vi "day 5 task 1.vi"() -> ()   [LabVIEW 2019]
panel:
  out "String":string
  out "Array 3":string[][](array[string])
  out "output array":string[][](array[string])
  out "Array":string[][](array[string])
  out "Array 2":string[][](array[string])
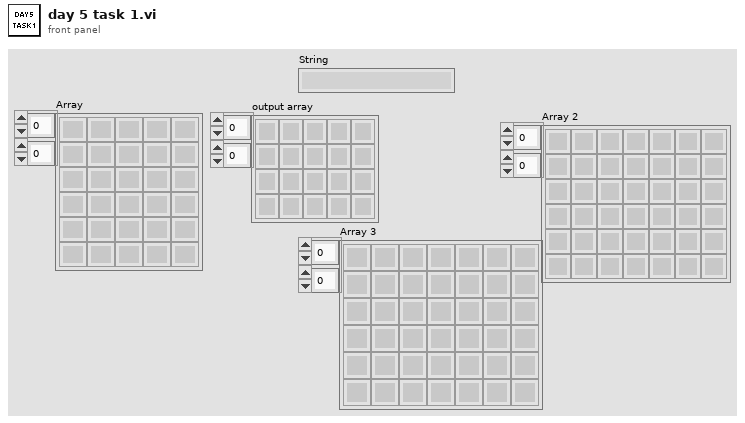
[diagram p1: front panel]
types:
  T1 = cluster{"no. crates to move":i32, "source col index":i32, "destination col index":i32}
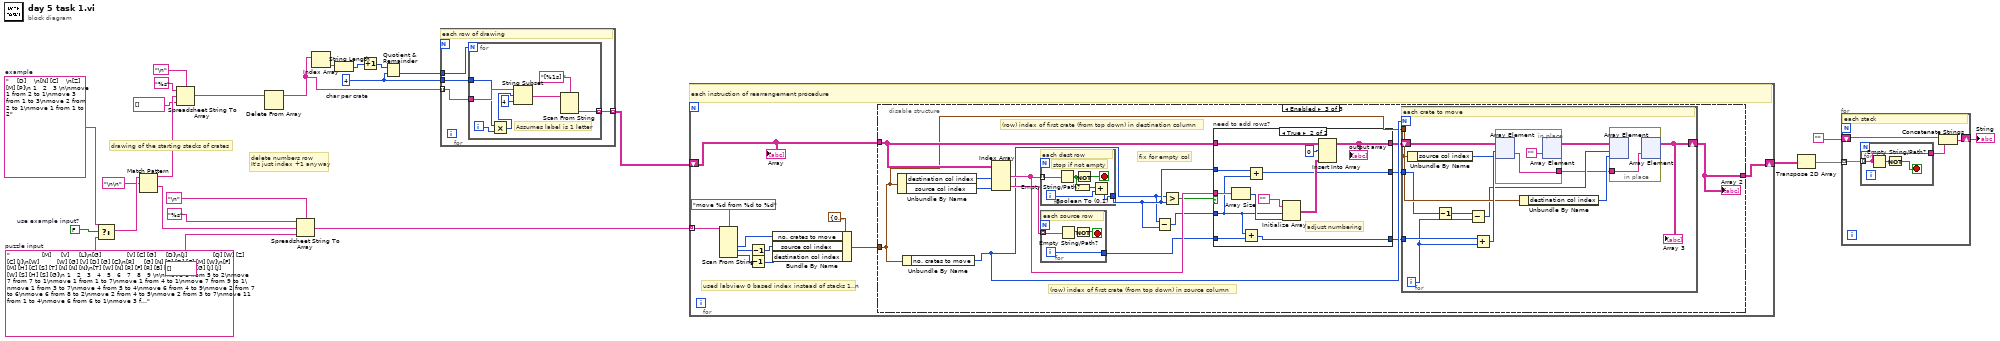
[diagram p0: block diagram]
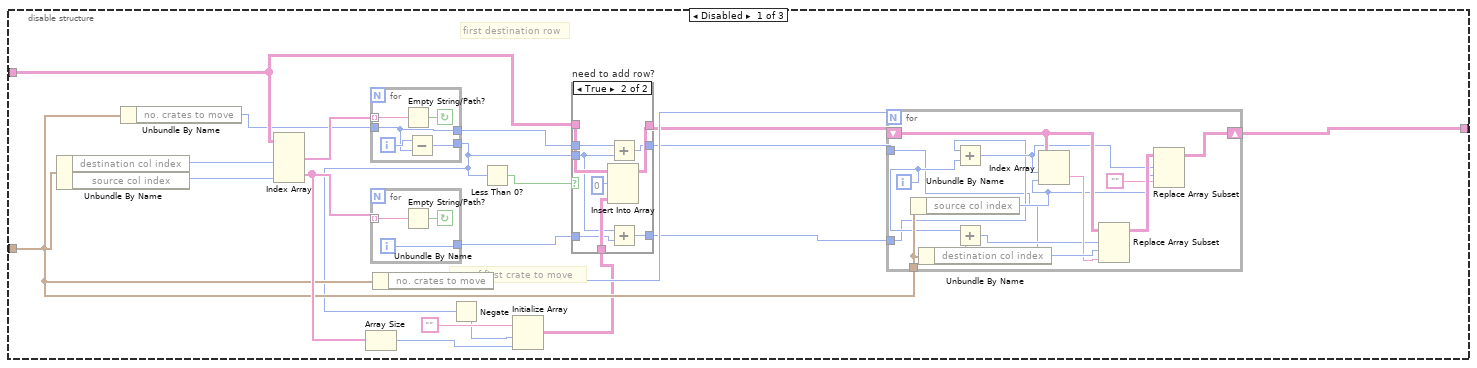
[diagram p2: hidden frame]
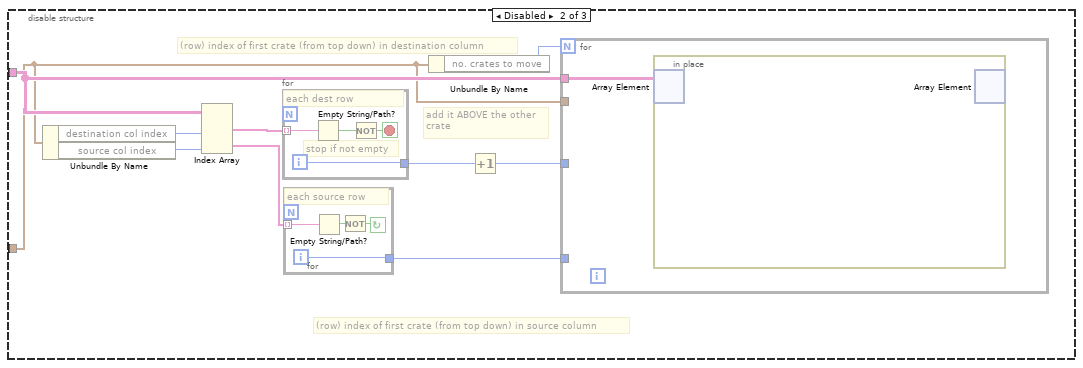
[diagram p4: hidden frame]
diagram:
  w11 = 4  # char per crate
  w21 = FALSE  # use example input?
  w22 = "                [M]     [V]     [L]\n[G]             [V] [C] [G]     [D]\n[J]             [Q] [W] [Z] [C] [J]\n[W]         [W] [G] [V] [D] [G] [C]\n[R]     [G] [N] [B] [D] [C] [M] [W]\n[F] [M] [H] [C] [S] [T] [N] [N] [N]\n[T] [W] [N] [R] [F] [R] [B] [J] [P]\n[Z] [G] [J] [J] [W] [S] [H] [S] [G]\n 1   2   3   4   5   6   7   8   9 \n\nmove 1 from 5 to 2\nmove 7 from 7 to 1\nmove 1 from 1 to 7\nmove 1 from 4 to 1\nmove 7 from 9 to 1\nmove 1 from 3 to 7\nmove 4 from 5 to 4\nmove 6 from 4 to 9\nmove 2 from 7 to 6\nmove 6 from 8 to 2\nmove 2 from 4 to 5\nmove 2 from 3 to 7\nmove 11 from 1 to 4\nmove 6 from 6 to 1\nmove 3 from 5 to 3\nmove 5 from 9 to 8\nmove 1 from 2 to 3\nmove 2 from 7 to 9\nmove 7 from 1 to 2\nmove 1 from 5 to 3\nmove 1 from 5 to 3\nmove 5 from 8 to 5\nmove 3 from 5 to 4\nmove 1 from 1 to 7\nmove 1 from 3 to 8\nmove 2 from 6 to 3\nmove 3 from 3 to 4\nmove 1 from 6 to 2\nmove 5 from 4 to 2\nmove 2 from 5 to 3\nmove 2 from 7 to 1\nmove 1 from 8 to 1\nmove 7 from 1 to 7\nmove 4 from 4 to 2\nmove 7 from 4 to 1\nmove 10 from 1 to 5\nmove 10 from 5 to 2\nmove 11 from 2 to 3\nmove 1 from 1 to 6\nmove 1 from 4 to 7\nmove 4 from 7 to 1\nmove 6 from 2 to 5\nmove 2 from 1 to 3\nmove 1 from 9 to 5\nmove 2 from 9 to 6\nmove 1 from 6 to 1\nmove 3 from 5 to 4\nmove 20 from 3 to 9\nmove 3 from 7 to 1\nmove 3 from 5 to 2\nmove 3 from 4 to 8\nmove 3 from 1 to 3\nmove 3 from 1 to 2\nmove 2 from 6 to 1\nmove 10 from 9 to 6\nmove 6 from 6 to 7\nmove 4 from 6 to 3\nmove 11 from 2 to 6\nmove 1 from 8 to 9\nmove 13 from 2 to 3\nmove 1 from 1 to 9\nmove 1 from 9 to 4\nmove 1 from 8 to 2\nmove 1 from 8 to 2\nmove 4 from 7 to 8\nmove 8 from 6 to 9\nmove 3 from 2 to 3\nmove 3 from 8 to 4\nmove 11 from 9 to 2\nmove 7 from 9 to 6\nmove 1 from 1 to 5\nmove 4 from 4 to 9\nmove 21 from 3 to 1\nmove 1 from 3 to 9\nmove 7 from 6 to 3\nmove 6 from 1 to 2\nmove 13 from 1 to 5\nmove 2 from 1 to 2\nmove 3 from 9 to 3\nmove 2 from 2 to 3\nmove 2 from 6 to 4\nmove 3 from 3 to 5\nmove 13 from 5 to 2\nmove 5 from 3 to 4\nmove 2 from 7 to 9\nmove 2 from 4 to 2\nmove 1 from 3 to 8\nmove 1 from 6 to 1\nmove 4 from 3 to 7\nmove 2 from 5 to 7\nmove 1 from 7 to 2\nmove 1 from 5 to 9\nmove 4 from 7 to 8\nmove 1 from 1 to 9\nmove 6 from 8 to 1\nmove 4 from 4 to 8\nmove 25 from 2 to 9\nmove 1 from 4 to 3\nmove 1 from 3 to 7\nmove 4 from 8 to 1\nmove 1 from 7 to 4\nmove 3 from 1 to 6\nmove 5 from 2 to 1\nmove 1 from 5 to 1\nmove 1 from 4 to 1\nmove 24 from 9 to 6\nmove 9 from 1 to 6\nmove 1 from 5 to 6\nmove 1 from 1 to 9\nmove 1 from 2 to 8\nmove 1 from 8 to 1\nmove 3 from 1 to 8\nmove 36 from 6 to 3\nmove 2 from 7 to 3\nmove 1 from 2 to 5\nmove 1 from 5 to 2\nmove 1 from 6 to 2\nmove 10 from 3 to 2\nmove 3 from 8 to 2\nmove 1 from 1 to 7\nmove 2 from 2 to 6\nmove 10 from 9 to 1\nmove 2 from 6 to 4\nmove 13 from 3 to 4\nmove 8 from 3 to 7\nmove 8 from 1 to 2\nmove 5 from 3 to 8\nmove 3 from 1 to 9\nmove 1 from 7 to 1\nmove 7 from 4 to 5\nmove 1 from 1 to 2\nmove 14 from 2 to 6\nmove 2 from 7 to 2\nmove 8 from 4 to 8\nmove 3 from 7 to 9\nmove 2 from 9 to 8\nmove 2 from 7 to 1\nmove 1 from 7 to 8\nmove 1 from 6 to 8\nmove 1 from 9 to 3\nmove 4 from 2 to 7\nmove 6 from 6 to 1\nmove 3 from 1 to 9\nmove 1 from 1 to 7\nmove 6 from 5 to 6\nmove 1 from 5 to 2\nmove 1 from 6 to 8\nmove 5 from 7 to 5\nmove 1 from 2 to 9\nmove 2 from 3 to 4\nmove 9 from 8 to 4\nmove 8 from 4 to 8\nmove 6 from 6 to 7\nmove 5 from 6 to 4\nmove 7 from 9 to 7\nmove 7 from 8 to 7\nmove 5 from 8 to 4\nmove 3 from 1 to 6\nmove 1 from 2 to 7\nmove 1 from 1 to 4\nmove 4 from 5 to 2\nmove 2 from 6 to 9\nmove 1 from 3 to 7\nmove 1 from 5 to 1\nmove 1 from 8 to 9\nmove 1 from 6 to 1\nmove 1 from 2 to 7\nmove 2 from 8 to 1\nmove 2 from 1 to 8\nmove 3 from 2 to 4\nmove 1 from 6 to 1\nmove 17 from 4 to 1\nmove 3 from 2 to 7\nmove 13 from 7 to 8\nmove 1 from 2 to 6\nmove 14 from 1 to 4\nmove 2 from 8 to 5\nmove 1 from 9 to 7\nmove 2 from 5 to 4\nmove 1 from 9 to 3\nmove 5 from 1 to 5\nmove 3 from 4 to 1\nmove 1 from 3 to 2\nmove 7 from 4 to 5\nmove 9 from 7 to 8\nmove 5 from 4 to 2\nmove 1 from 1 to 3\nmove 1 from 9 to 2\nmove 15 from 8 to 6\nmove 1 from 3 to 7\nmove 11 from 6 to 5\nmove 1 from 4 to 8\nmove 3 from 1 to 7\nmove 5 from 7 to 5\nmove 27 from 5 to 1\nmove 8 from 8 to 4\nmove 1 from 2 to 6\nmove 3 from 6 to 1\nmove 9 from 1 to 5\nmove 5 from 5 to 7\nmove 2 from 2 to 1\nmove 2 from 5 to 4\nmove 6 from 7 to 6\nmove 1 from 5 to 2\nmove 1 from 7 to 8\nmove 4 from 6 to 8\nmove 5 from 6 to 3\nmove 1 from 7 to 1\nmove 5 from 4 to 3\nmove 6 from 8 to 2\nmove 1 from 7 to 8\nmove 2 from 8 to 9\nmove 10 from 3 to 5\nmove 9 from 5 to 2\nmove 3 from 4 to 8\nmove 1 from 5 to 7\nmove 2 from 9 to 7\nmove 2 from 8 to 3\nmove 1 from 3 to 8\nmove 19 from 1 to 7\nmove 4 from 2 to 7\nmove 2 from 4 to 3\nmove 3 from 3 to 2\nmove 2 from 8 to 3\nmove 2 from 5 to 8\nmove 1 from 2 to 3\nmove 2 from 8 to 3\nmove 5 from 2 to 5\nmove 9 from 7 to 5\nmove 13 from 5 to 9\nmove 7 from 2 to 6\nmove 2 from 6 to 9\nmove 1 from 2 to 1\nmove 5 from 6 to 7\nmove 1 from 5 to 7\nmove 6 from 1 to 2\nmove 5 from 3 to 6\nmove 6 from 7 to 2\nmove 3 from 6 to 4\nmove 3 from 7 to 4\nmove 12 from 7 to 6\nmove 5 from 4 to 1\nmove 2 from 7 to 4\nmove 3 from 4 to 6\nmove 16 from 6 to 3\nmove 4 from 1 to 4\nmove 1 from 1 to 9\nmove 3 from 9 to 2\nmove 1 from 4 to 6\nmove 9 from 3 to 7\nmove 2 from 6 to 3\nmove 3 from 3 to 9\nmove 15 from 2 to 7\nmove 19 from 7 to 4\nmove 15 from 9 to 2\nmove 16 from 2 to 8\nmove 6 from 3 to 5\nmove 4 from 7 to 5\nmove 15 from 8 to 7\nmove 19 from 4 to 2\nmove 1 from 8 to 3\nmove 16 from 2 to 1\nmove 9 from 7 to 6\nmove 7 from 2 to 8\nmove 2 from 2 to 7\nmove 1 from 9 to 5\nmove 1 from 3 to 4\nmove 6 from 1 to 2\nmove 8 from 5 to 1\nmove 1 from 5 to 1\nmove 18 from 1 to 8\nmove 7 from 7 to 5\nmove 7 from 5 to 3\nmove 4 from 3 to 6\nmove 13 from 8 to 5\nmove 12 from 8 to 1\nmove 5 from 1 to 6\nmove 15 from 5 to 4\nmove 1 from 1 to 6\nmove 12 from 6 to 3\nmove 8 from 3 to 4\nmove 2 from 7 to 3\nmove 9 from 3 to 1\nmove 5 from 2 to 9\nmove 16 from 4 to 3\nmove 10 from 1 to 3\nmove 2 from 1 to 5\nmove 1 from 3 to 1\nmove 5 from 6 to 1\nmove 4 from 9 to 3\nmove 1 from 2 to 8\nmove 1 from 8 to 1\nmove 1 from 9 to 8\nmove 2 from 5 to 9\nmove 9 from 4 to 1\nmove 3 from 1 to 3\nmove 2 from 6 to 8\nmove 3 from 8 to 5\nmove 2 from 1 to 5\nmove 2 from 9 to 8\nmove 1 from 8 to 6\nmove 2 from 5 to 3\nmove 19 from 3 to 1\nmove 2 from 4 to 2\nmove 1 from 5 to 6\nmove 2 from 2 to 3\nmove 1 from 8 to 6\nmove 8 from 3 to 9\nmove 6 from 3 to 7\nmove 2 from 6 to 2\nmove 1 from 6 to 1\nmove 1 from 1 to 8\nmove 1 from 8 to 9\nmove 1 from 7 to 3\nmove 19 from 1 to 5\nmove 21 from 5 to 2\nmove 13 from 2 to 6\nmove 13 from 1 to 8\nmove 7 from 9 to 7\nmove 2 from 9 to 2\nmove 10 from 8 to 3\nmove 1 from 1 to 6\nmove 10 from 2 to 4\nmove 11 from 3 to 5\nmove 8 from 5 to 6\nmove 1 from 3 to 7\nmove 2 from 8 to 6\nmove 2 from 2 to 8\nmove 3 from 7 to 6\nmove 2 from 8 to 6\nmove 1 from 1 to 2\nmove 24 from 6 to 5\nmove 2 from 3 to 8\nmove 1 from 8 to 6\nmove 7 from 7 to 9\nmove 4 from 6 to 9\nmove 1 from 8 to 9\nmove 21 from 5 to 9\nmove 2 from 7 to 2\nmove 1 from 8 to 5\nmove 1 from 7 to 3\nmove 12 from 9 to 6\nmove 6 from 6 to 3\nmove 12 from 9 to 4\nmove 4 from 5 to 6\nmove 13 from 4 to 2\nmove 8 from 4 to 8\nmove 10 from 6 to 8\nmove 11 from 8 to 9\nmove 4 from 8 to 4\nmove 2 from 4 to 3\nmove 8 from 3 to 8\nmove 2 from 6 to 8\nmove 1 from 3 to 8\nmove 6 from 2 to 4\nmove 1 from 4 to 8\nmove 1 from 9 to 7\nmove 13 from 8 to 4\nmove 1 from 7 to 1\nmove 1 from 1 to 4\nmove 8 from 4 to 7\nmove 3 from 5 to 7\nmove 19 from 9 to 7\nmove 3 from 2 to 7\nmove 1 from 8 to 2\nmove 13 from 7 to 6\nmove 1 from 2 to 4\nmove 4 from 6 to 2\nmove 1 from 8 to 3\nmove 7 from 6 to 8\nmove 1 from 6 to 2\nmove 1 from 2 to 7\nmove 9 from 2 to 3\nmove 1 from 6 to 2\nmove 21 from 7 to 5\nmove 9 from 5 to 3\nmove 19 from 3 to 9\nmove 5 from 8 to 5\nmove 2 from 2 to 1\nmove 2 from 1 to 8\nmove 6 from 4 to 5\nmove 3 from 8 to 7\nmove 15 from 9 to 2\nmove 2 from 2 to 5\nmove 3 from 9 to 6\nmove 5 from 4 to 5\nmove 11 from 2 to 6\nmove 1 from 8 to 6\nmove 1 from 9 to 5\nmove 1 from 7 to 3\nmove 6 from 5 to 6\nmove 1 from 4 to 6\nmove 1 from 3 to 4\nmove 13 from 5 to 2\nmove 16 from 6 to 9\nmove 4 from 4 to 5\nmove 2 from 6 to 2\nmove 2 from 6 to 4\nmove 2 from 4 to 5\nmove 2 from 7 to 8\nmove 2 from 6 to 3\nmove 2 from 5 to 8\nmove 14 from 5 to 7\nmove 4 from 8 to 1\nmove 4 from 1 to 6\nmove 1 from 3 to 9\nmove 1 from 6 to 1\nmove 2 from 7 to 3\nmove 2 from 3 to 7\nmove 2 from 5 to 2\nmove 9 from 9 to 2\nmove 13 from 7 to 3\nmove 12 from 3 to 9\nmove 2 from 6 to 8\nmove 14 from 2 to 9\nmove 2 from 8 to 9\nmove 10 from 2 to 1\nmove 1 from 7 to 4\nmove 2 from 3 to 8\nmove 4 from 2 to 1\nmove 1 from 8 to 3\nmove 1 from 2 to 6\nmove 1 from 8 to 3\nmove 4 from 9 to 4\nmove 1 from 3 to 5\nmove 1 from 5 to 1\nmove 1 from 3 to 9\nmove 12 from 1 to 8\nmove 10 from 8 to 5\nmove 7 from 5 to 6\nmove 1 from 1 to 9\nmove 3 from 5 to 1\nmove 1 from 1 to 3\nmove 16 from 9 to 7\nmove 4 from 4 to 3\nmove 1 from 4 to 9\nmove 15 from 7 to 8\nmove 15 from 9 to 1\nmove 8 from 1 to 6\nmove 1 from 9 to 3\nmove 17 from 6 to 2\nmove 1 from 9 to 1\nmove 15 from 2 to 7\nmove 14 from 8 to 9\nmove 12 from 7 to 9\nmove 12 from 9 to 3\nmove 3 from 7 to 9\nmove 1 from 7 to 4\nmove 7 from 9 to 6\nmove 1 from 4 to 6\nmove 11 from 9 to 6\nmove 2 from 1 to 2\nmove 18 from 6 to 4\nmove 4 from 2 to 7\nmove 2 from 7 to 3\nmove 2 from 7 to 8\nmove 4 from 1 to 5\nmove 1 from 9 to 2\nmove 2 from 5 to 4\nmove 5 from 1 to 3\nmove 2 from 3 to 7\nmove 2 from 3 to 9\nmove 1 from 6 to 7\nmove 1 from 2 to 9\nmove 2 from 8 to 1\nmove 3 from 1 to 3\nmove 2 from 5 to 8\nmove 2 from 3 to 5\nmove 1 from 5 to 2\nmove 1 from 1 to 3\nmove 1 from 9 to 2\nmove 1 from 9 to 1\nmove 3 from 7 to 6\nmove 1 from 1 to 9\nmove 2 from 8 to 9\nmove 1 from 2 to 3\nmove 2 from 8 to 2\nmove 2 from 6 to 5\nmove 1 from 8 to 5\nmove 3 from 2 to 5\nmove 3 from 4 to 8\nmove 1 from 8 to 2\nmove 3 from 9 to 7\nmove 3 from 7 to 1\nmove 1 from 9 to 6\nmove 3 from 1 to 2\nmove 2 from 8 to 7\nmove 2 from 7 to 9\nmove 2 from 6 to 5\nmove 3 from 5 to 3\nmove 1 from 2 to 5\nmove 3 from 2 to 7\nmove 2 from 5 to 6\nmove 15 from 4 to 9\nmove 1 from 3 to 1\nmove 25 from 3 to 4\nmove 3 from 7 to 3\nmove 5 from 9 to 5\nmove 10 from 9 to 5\nmove 9 from 5 to 1\nmove 5 from 5 to 2\nmove 1 from 6 to 7\nmove 5 from 5 to 8"  # puzzle input
  w23 = "    [D]    \n[N] [C]    \n[Z] [M] [P]\n 1   2   3 \n\nmove 1 from 2 to 1\nmove 3 from 1 to 3\nmove 2 from 2 to 1\nmove 1 from 1 to 2"  # example
  # "delete numbers row\nIt's just index +1 anyway"
  # "drawing of the starting stacks of crates"
  n1 = Select(t=w23, s=w21, f=w22) -> (s? t:f=w19:string)
  n2 = Match Pattern(string=w19, regular expression="\n\n" ("example")) -> (before substring=w14:string, after substring=w17:string)  [unwired: 1 in, 2 out]
  n3 = Spreadsheet String To Array(delimiter (Tab)="\n", format string="%s", spreadsheet string=w14, array type (2D Dbl)=string[] []) -> (array=w9:string[])
  n4 = Delete From Array(array=w9) -> (array with subset deleted=w10:string[])  [unwired: 2 in, 1 out]
  n5 = Spreadsheet String To Array(delimiter (Tab)="\n", format string="%s", spreadsheet string=w17, array type (2D Dbl)=string[] []) -> (array=w20:string[])
  n6 = Index Array(array=w10) -> (element=w13:string)  [unwired: 1 in]
  n7 = String Length(string=w13) -> (length=w1:i32)
  n8 = Increment(x=w1) -> (x+1=w2:i32)
  n9 = Quotient & Remainder(x=w2, y=w11) -> (floor(x/y)=w3:i32)  [unwired: 1 out]
  n10 = for {
    tunnel: w10 -> [w30] mode=indexing
    tunnel: w11 -> [w28]
    tunnel: [w29] -> w8 mode=indexing
    tunnel: w3 -> [w27]
    # "each row of drawing"
    n11 = for {
      N: w27 -> [_]
      tunnel: w28 -> [w34]
      tunnel: w30 -> [w38]
      tunnel: [w31] -> w29 mode=indexing
      i -> [w35]
      # "Assumes label is 1 letter"
      n12 = Multiply(x=w34, y=w35) -> (x*y=w36:i32)
      n13 = String Subset(string=w38, offset (0)=w36, length (rest)=4 ("length (rest)")) -> (substring=w32:string)
      n14 = Scan From String(format string="[%1s] ", input string=w32) -> (output 1=w31:string)  [unwired: 3 in, 3 out]
    }
  }
  n15 = for {
    tunnel: w20 -> [w49] mode=indexing
    shift-right: [w39] -> w7
    shift-left: w8 -> [w41]
    # "used labview 0 based index instead of stacks 1..n"
    # "each instruction of rearrangement procedure"
    n16 = Scan From String(format string="move %d from %d to %d", input string=w49) -> (output 1=w44:i32, output 2=w47:i32, output 3=w46:i32)  [unwired: 5 in, 3 out]
    n17 = Decrement(x=w46) -> (x-1=w42:i32)
    n18 = Decrement(x=w47) -> (x-1=w43:i32)
    n19 = Bundle By Name(cluster=T1 {"no. crates to move"=0, "source col index"=0, "destination col index"=0}, "no. crates to move"=w44, "source col index"=w43, "destination col index"=w42) -> (w40:T1)
    n20 = disable-structure shown="Enabled" {
      disable-tunnel: [w65 _ w122] -> w39
      disable-tunnel: w41 -> [w64 w104 w131]
      disable-tunnel: w40 -> [w55 w103 w123]
      frame Disabled {
        # "first destination row"
        # "row of first crate to move"
        n21 = Unbundle By Name(w55) -> ("destination col index"=w69:i32, "source col index"=w68:i32)
        n22 = Unbundle By Name(w55) -> ("no. crates to move"=w56:i32)
        n23 = Index Array(array=w64, index (col) #1=w69, index (col) #2=w68) -> (element #1=w66:string[], element #2=w61:string[])  [unwired: 2 in]
        n24 = Array Size(array=w61) -> (size(s)=w53:i32)
        n25 = for {
          tunnel: w66 -> [w102] mode=indexing
          tunnel: [w99] -> w50
          tunnel: w56 -> [w98]
          tunnel: [w98] -> w51
          i -> [w100]
          stop <- w101 continue-if-true
          n26 = Empty String/Path?(string/path=w102) -> (empty?=w101:bool)
          n27 = Subtract(x=w100, y=w98) -> (x-y=w99:i32)
        }
        n28 = for {
          tunnel: w61 -> [w97] mode=indexing
          tunnel: [w95] -> w58
          i -> [w95]
          stop <- w96 continue-if-true
          n29 = Empty String/Path?(string/path=w97) -> (empty?=w96:bool)
        }
        n30 = Unbundle By Name(w55) -> ("no. crates to move"=w67:i32)
        n31 = Negate(x=w50) -> (-x=w54:i32)
        n32 = Less Than 0?(x=w50) -> (x < 0?=w57:bool)
        n33 = Initialize Array("", w54, w53) -> (w52:string[][])
        n34 = case "need to add row?" shown="True" w57 {
          tunnel: w64 -> [w85 w94]
          tunnel: [w85 w93] -> w63
          tunnel: w52 -> [_ w92]
          tunnel: w51 -> [w84 w88]
          tunnel: [w84 w87] -> w60
          tunnel: [w83 w91] -> w59
          tunnel: w58 -> [w83 w90]
          tunnel: w50 -> [_ w86]
          frame False {
          }
          frame True {
            n35 = Insert Into Array(array=w94, index (row)=0, new element=w92) -> (w93:string[][])  [unwired: 1 in]
            n36 = Add(x=w88, y=w86) -> (x+y=w87:i32)
            n37 = Add(x=w86, y=w90) -> (x+y=w91:i32)
          }
        }
        n38 = for {
          N: w67 -> [_]
          tunnel: w60 -> [w70]
          tunnel: w59 -> [w71]
          tunnel: w55 -> [w82]
          shift-right: [w75] -> w65
          shift-left: w63 -> [w80]
          i -> [w72]
          n39 = Unbundle By Name(w82) -> ("source col index"=w77:i32)
          n40 = Unbundle By Name(w82) -> ("destination col index"=w79:i32)
          n41 = Add(x=w71, y=w72) -> (x+y=w73:i32)
          n42 = Add(x=w72, y=w70) -> (x+y=w74:i32)
          n43 = Index Array(array=w80, index (row)=w73, index (col)=w77) -> (element=w78:string)
          n44 = Replace Array Subset(array=w80, new element=w78, index (row)=w74, index (col)=w79) -> (w81:string[][])
          n45 = Replace Array Subset(array=w81, new element="", index (row)=w73, index (col)=w77) -> (w75:string[][])
        }
      }
      frame Disabled {
        # "add it ABOVE the other\ncrate"
        # "(row) index of first crate (from top down) in source column"
        # "(row) index of first crate (from top down) in destination column"
        n46 = Unbundle By Name(w103) -> ("destination col index"=w111:i32, "source col index"=w112:i32)
        n47 = Index Array(array=w104, index (col) #1=w111, index (col) #2=w112) -> (element #1=w109:string[], element #2=w110:string[])  [unwired: 2 in]
        n48 = for {
          tunnel: [w121] -> w106
          tunnel: w109 -> [w120] mode=indexing
          i -> [w121]
          stop <- w119 stop-if-true
          # "stop if not empty"
          # "each dest row"
          n49 = Empty String/Path?(string/path=w120) -> (empty?=w118:bool)
          n50 = Not(x=w118) -> (.not. x?=w119:bool)
        }
        n51 = for {
          tunnel: [w117] -> w107
          tunnel: w110 -> [w116] mode=indexing
          i -> [w117]
          stop <- w115 continue-if-true
          # "each source row"
          n52 = Empty String/Path?(string/path=w116) -> (empty?=w114:bool)
          n53 = Not(x=w114) -> (.not. x?=w115:bool)
        }
        n54 = Unbundle By Name(w103) -> ("no. crates to move"=w108:i32)
        n55 = Increment(x=w106) -> (x+1=w105:i32)
        n56 = for {
          N: w108 -> [_]
          tunnel: w107 -> [_]
          tunnel: w105 -> [_]
          tunnel: w104 -> [w113]
          tunnel: w103 -> [_]
          n57 = in-place {
            n58 = in-place-array #1(w113) -> ()  [unwired: 2 in, 1 out]
            n59 = in-place-array #1() -> ()  [unwired: 1 in, 3 out]
          }
        }
      }
      frame Enabled {
        # "fix for empty col"
        # "(row) index of first crate (from top down) in source column"
        # "(row) index of first crate (from top down) in destination column"
        n60 = Unbundle By Name(w123) -> ("destination col index"=w135:i32, "source col index"=w136:i32)
        n61 = Unbundle By Name(w123) -> ("no. crates to move"=w128:i32)
        n62 = Index Array(array=w131, index (col) #1=w135, index (col) #2=w136) -> (element #1=w133:string[], element #2=w134:string[])  [unwired: 2 in]
        n63 = for {
          tunnel: [w172] -> w130
          tunnel: w133 -> [w177] mode=indexing
          i -> [w174]
          stop <- w176 stop-if-true
          # "stop if not empty"
          # "each dest row"
          n64 = Empty String/Path?(string/path=w177) -> (empty?=w173:bool)
          n65 = Boolean To (0,1)(Boolean=w173) -> (0, 1=w175:i16)
          n66 = Not(x=w173) -> (.not. x?=w176:bool)
          n67 = Add(x=w175, y=w174) -> (x+y=w172:i32)
        }
        n68 = for {
          tunnel: [w171] -> w129
          tunnel: w134 -> [w170] mode=indexing
          i -> [w171]
          stop <- w169 stop-if-true
          # "each source row"
          n69 = Empty String/Path?(string/path=w170) -> (empty?=w168:bool)
          n70 = Not(x=w168) -> (.not. x?=w169:bool)
        }
        n71 = Subtract(x=w128, y=w130) -> (x-y=w132:i32)
        n72 = Greater?(x=w128, y=w130) -> (0:w126:bool)
        n73 = case "need to add rows?" shown="True" w126 {
          tunnel: w133 -> [_ w167]
          tunnel: w132 -> [_ w158]
          tunnel: w131 -> [w153 w162]
          tunnel: [w153 w161] -> w127
          tunnel: [w155 w156] -> w124
          tunnel: w130 -> [w155 w160]
          tunnel: [w154 w157] -> w125
          tunnel: w129 -> [w154 w159]
          frame False {
          }
          frame True {
            # "adjust numbering"
            n74 = Array Size(array=w167) -> (size(s)=w165:i32)
            n75 = Add(x=w158, y=w159) -> (x+y=w157:i32)
            n76 = Add(x=w160, y=w158) -> (x+y=w156:i32)
            n77 = Initialize Array("", w158, w165) -> (w163:string[][])
            n78 = Insert Into Array(array=w162, index (row)=0, new element=w163) -> (w161:string[][])  [unwired: 1 in]
            "output array" <- w161
          }
        }
        n79 = for {
          N: w128 -> [_]
          tunnel: w125 -> [w147]
          tunnel: w124 -> [w141]
          tunnel: w123 -> [w144]
          shift-right: [w138] -> w122
          shift-left: w127 -> [w149]
          i -> [w142]
          # "each crate to move"
          n80 = Unbundle By Name(w144) -> ("source col index"=w145:i32)
          n81 = Decrement(x=w141) -> (x-1=w137:i32)
          n82 = Subtract(x=w137, y=w142) -> (x-y=w140:i32)
          n83 = Add(x=w147, y=w142) -> (x+y=w146:i32)
          n84 = in-place {
            in-place-border: [w152] -> w139
            n85 = in-place-array #2(w149, w146, w145) -> (w152:string)
            n86 = in-place-array #2("") -> (w148:string[][])  [unwired: 2 out]
          }
          n87 = Unbundle By Name(w144) -> ("destination col index"=w143:i32)
          n88 = in-place {
            in-place-border: w139 -> [w150]
            n89 = in-place-array #3(w148, w140, w143) -> ()  [unwired: 1 out]
            n90 = in-place-array #3(w150) -> (w138:string[][])  [unwired: 2 out]
          }
          "Array 3" <- w138
        }
        "Array 2" <- w122
      }
    }
    "Array" <- w41
  }
  n91 = Transpose 2D Array(2D array=w7) -> (transposed array=w6:string[][])
  n92 = for {
    tunnel: w6 -> [w181] mode=indexing
    shift-right: [w180] -> w4
    shift-left: "" -> [w179]
    # "each stack"
    n93 = for {
      tunnel: w181 -> [w182] mode=indexing
      tunnel: [w182] -> w178
      stop <- w183 stop-if-true
      n94 = Empty String/Path?(string/path=w182) -> (empty?=w184:bool)
      n95 = Not(x=w184) -> (.not. x?=w183:bool)
    }
    n96 = Concatenate Strings(w179, w178) -> (w180:string)
  }
  "String" <- w4
